vi "myRIO_BRig_RT_dataCurrent_nRewTrials.vi"() -> (2 "output_nRewTrials":i32)   [LabVIEW 2014]
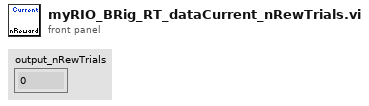
[diagram p1: front panel]
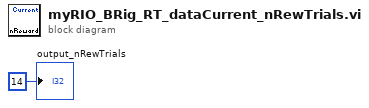
[diagram p0: block diagram]
diagram:
  "output_nRewTrials" <- 14 ("output_iBlock")
